vi "ReCalc_V0.14.vi"(3 "Berechnen":bool, 4 "Datenspeicher":T2) -> ()   [LabVIEW 2014]
uses:
  <vilib>/Utility/miscctls.llb/LVPointTypeDef.ctl
  <vilib>/Analysis/NI_AALBase.lvlib
  <vilib>/Analysis/NI_AALPro.lvlib
  <vilib>/Utility/xml.llb/Read From XML File(string).vi
  <vilib>/Analysis/3filter.llb/IIR Filter (DBL).vi
  <vilib>/Utility/xml.llb/Write to XML File(string).vi
panel:
  out "Fahrzeugdaten":string
  out "Überlagerung":bool
  in  "Überlagern":bool
  out "Übersetzung ermitteln aus":T1(ring)
  in  "Speichern":bool
  out "Reifenumfang [m]":dbl=1.222
  out "Getriebe [1:]":dbl=5.343
  out "Zündung [Imp/U]":u8=1
  out "Rolle [Inkr/U]":u16=200
  out "Luftdruck [mbar]":dbl=1013.0
  out "Luftfeuchtigkeit [%]":dbl=50.0
  out "Lufttemperatur [°C]":dbl=20.0
  in  "Stopp":bool
  in  "Rollenträgheit [kgm²]":dbl=0.402
  in  "Polynom":u8=15
  in  "Gl. Mittelwert":u8=35
  in  "Differenzenquotient":u8=12
  in  "n vom Gas [1/min]":dbl=5000.0
  out "Rollenumfang [m]":dbl=0.613 format="%.3f"
  out "Datum, Zeit":string
  out "Untersetzung aus:":dbl=2.68 format="%.2f"
  in  "Drucken":bool
  out "Pmax":string
  out "Ergebnis":string
  out "XY-Graph":cluster{dbl[], dbl[]}[](graph)
  in  "Öffnen":bool
  out "korr":dbl
  out "[s]":dbl=5.0
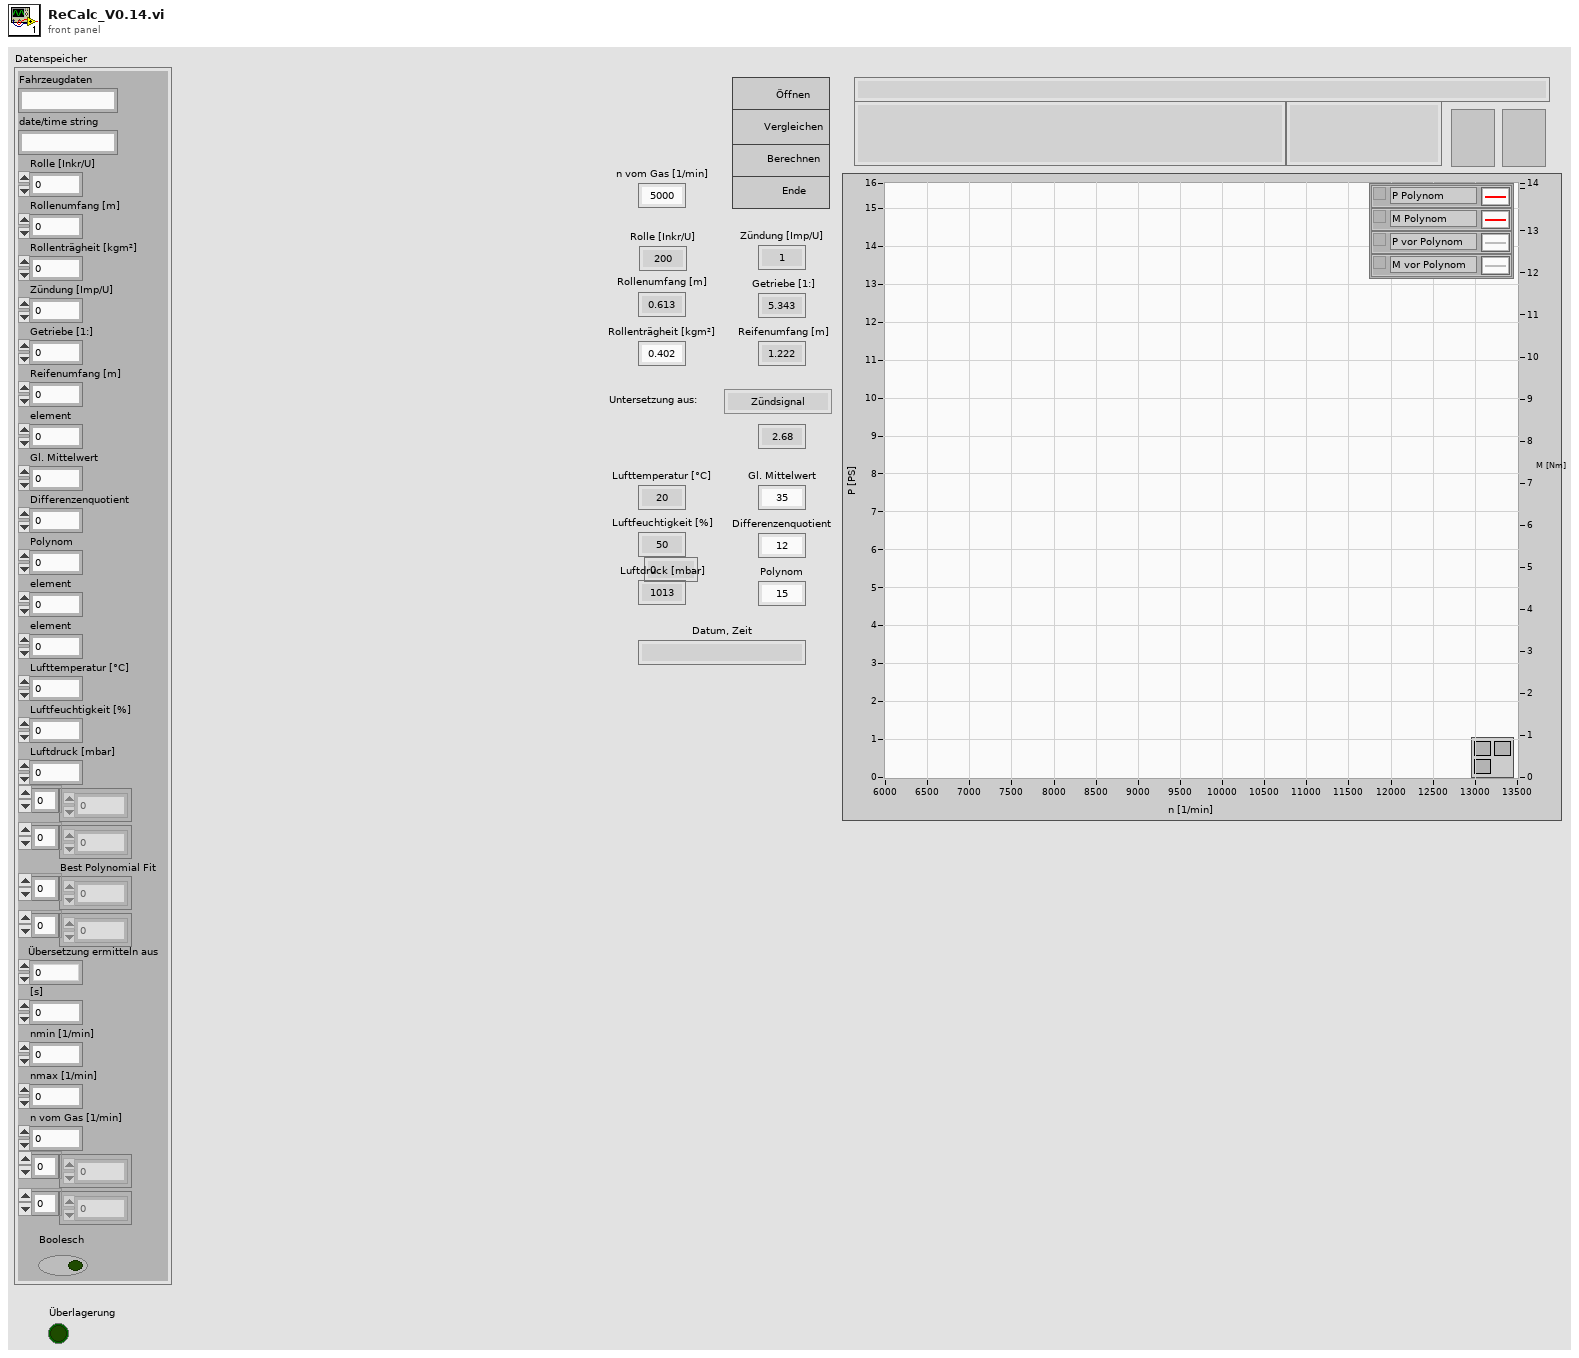
[diagram p1: front panel]
types:
  T1 = enum8{"Zündsignal", "Getriebe & Reifen", "nKuWe / nRolle :"}
  T2 = cluster{"Fahrzeugdaten":string, "date/time string":string, "Rolle [Inkr/U]":u16, "Rollenumfang [m]":dbl, "Rollenträgheit [kgm²]":dbl, "Zündung [Imp/U]":u8, "Getriebe [1:]":dbl, "Reifenumfang [m] ":dbl, "element":dbl, "Gl. Mittelwert":u8, "Differenzenquotient":u8, "Polynom":u8, "element":dbl, "element":dbl, "Lufttemperatur [°C]":dbl, "Luftfeuchtigkeit [%]":dbl, "Luftdruck [mbar]":dbl, dbl[], dbl[], "Best Polynomial Fit":dbl[], dbl[], "Übersetzung ermitteln aus":u8, "[s]":dbl, "nmin [1/min]":dbl, "nmax [1/min]":dbl, "n vom Gas [1/min]":dbl, dbl[], i32[], "Boolesch":bool}
  T3 = typedef "LVPointTypeDef.ctl" = cluster{"Horizontal":i16, "Vertical":i16}
  T4 = enum16{"Kleinste Quadrate", "Kleinestes absolutes Reiduum", "Biquadrat"}
  T5 = enum8{"Enabled", "Disabled", "Disabled and Grayed Out"}
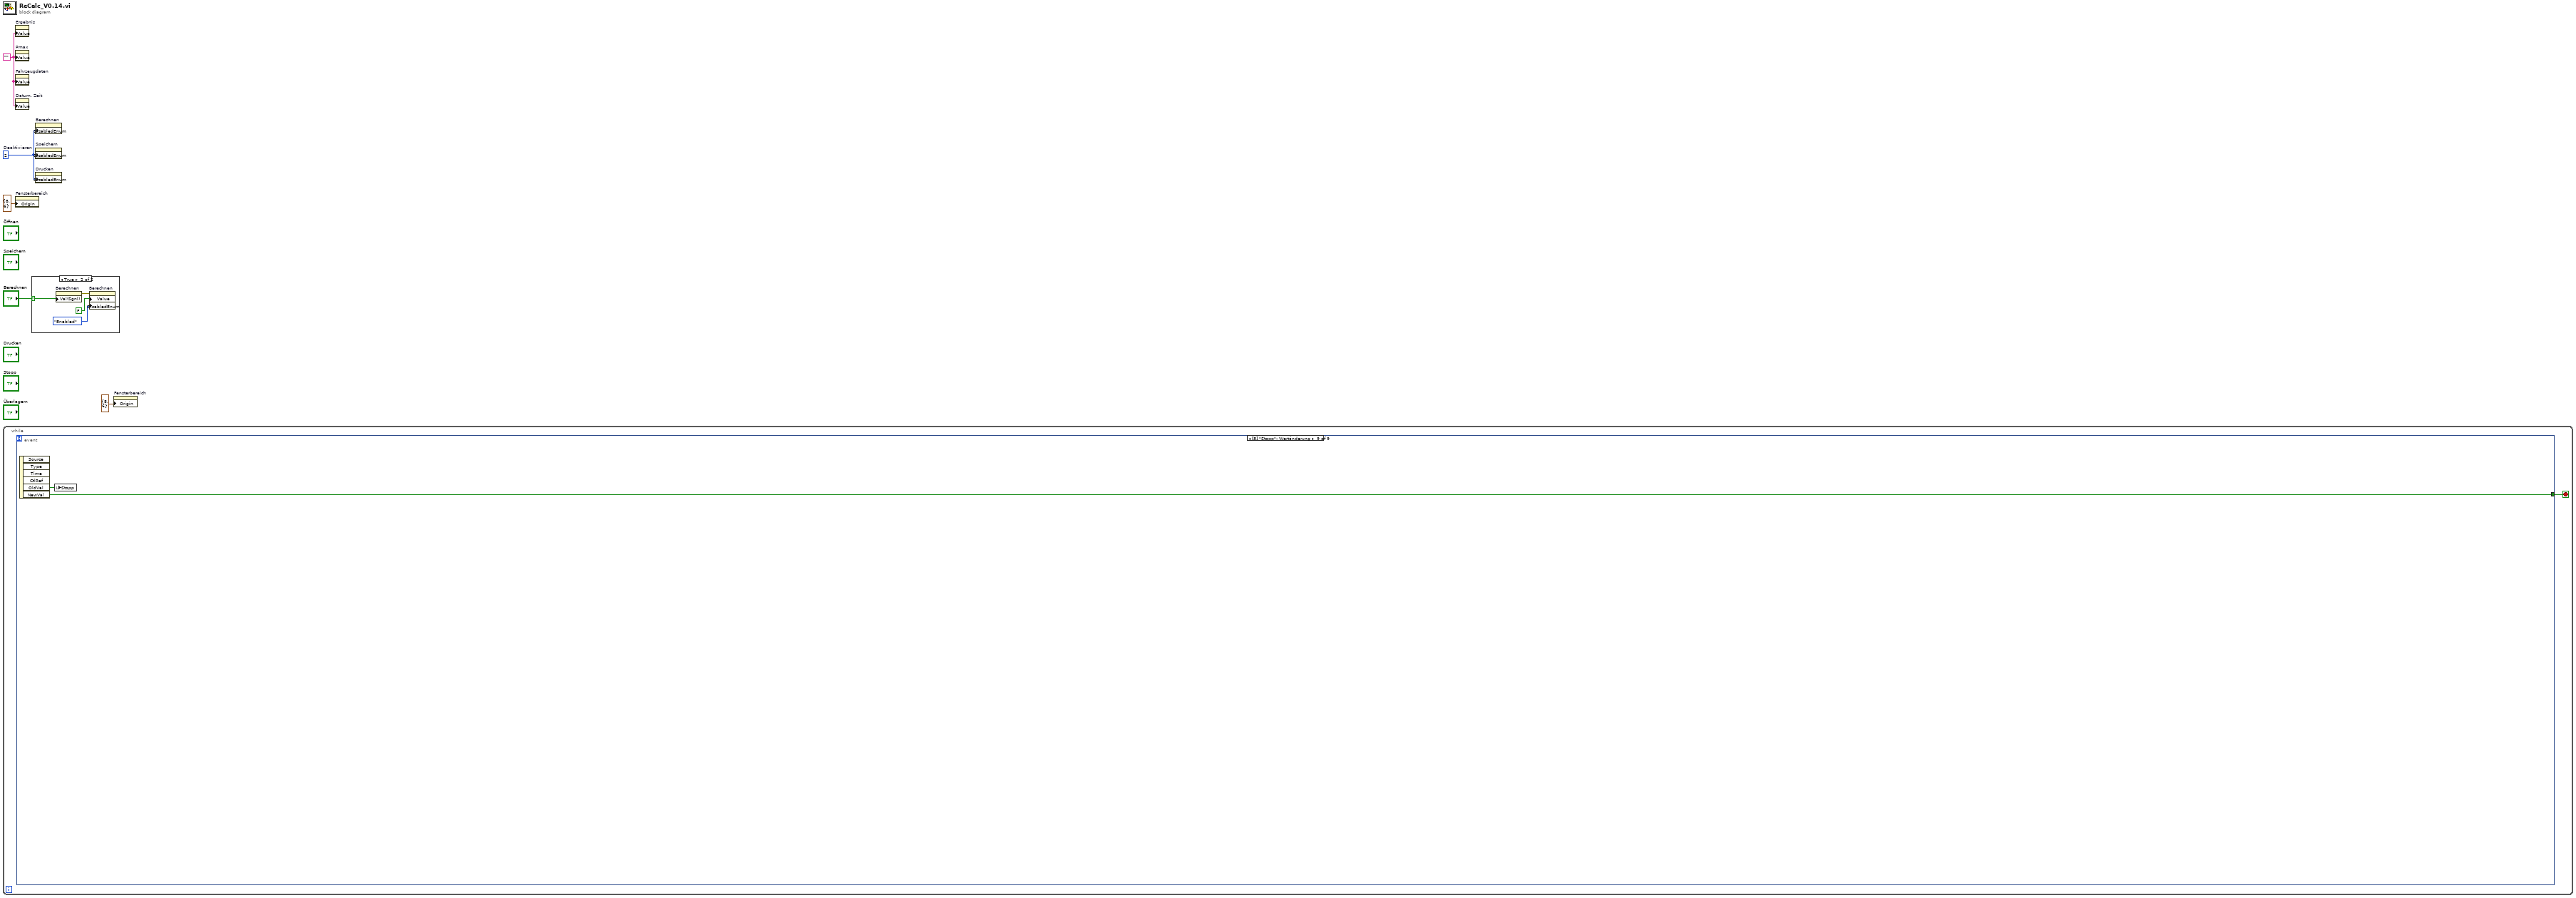
[diagram p0: block diagram]
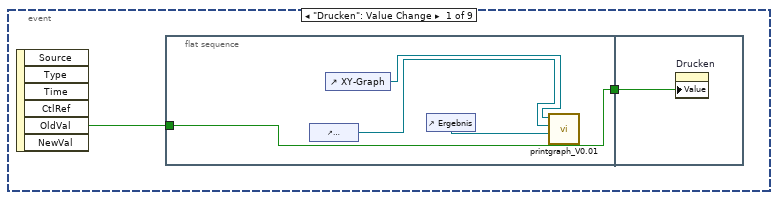
[diagram p3: hidden frame]
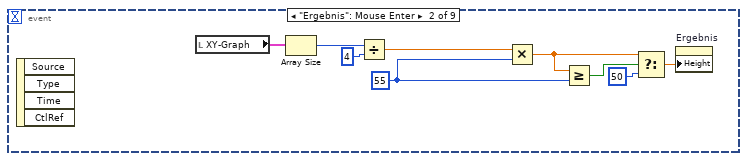
[diagram p4: hidden frame]
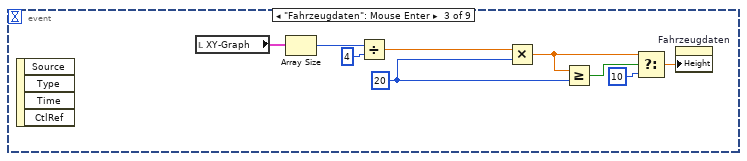
[diagram p5: hidden frame]
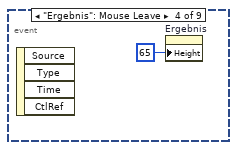
[diagram p6: hidden frame]
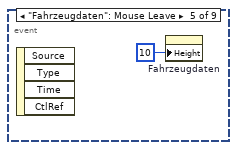
[diagram p7: hidden frame]
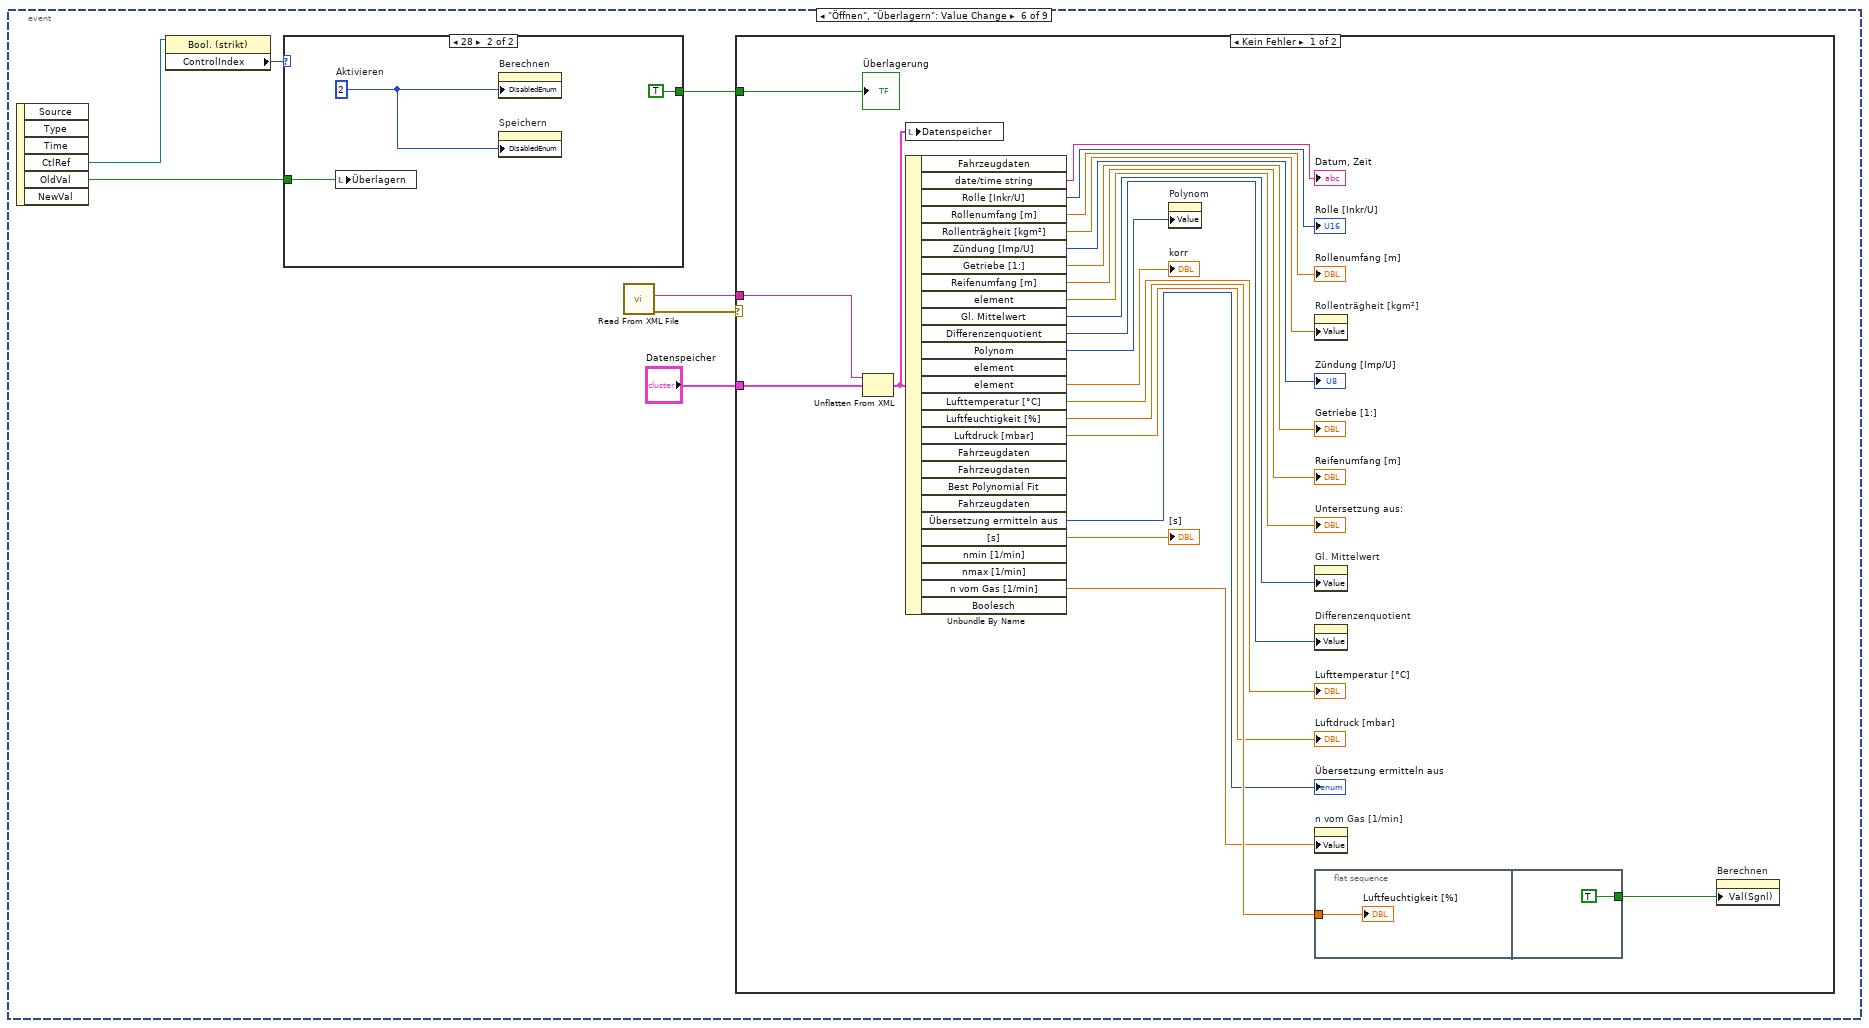
[diagram p8: hidden frame]
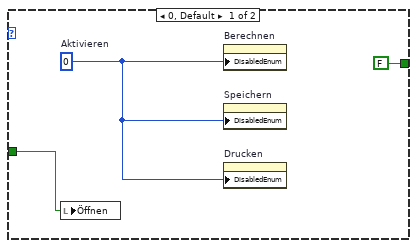
[diagram p9: hidden frame]
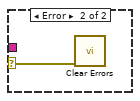
[diagram p10: hidden frame]
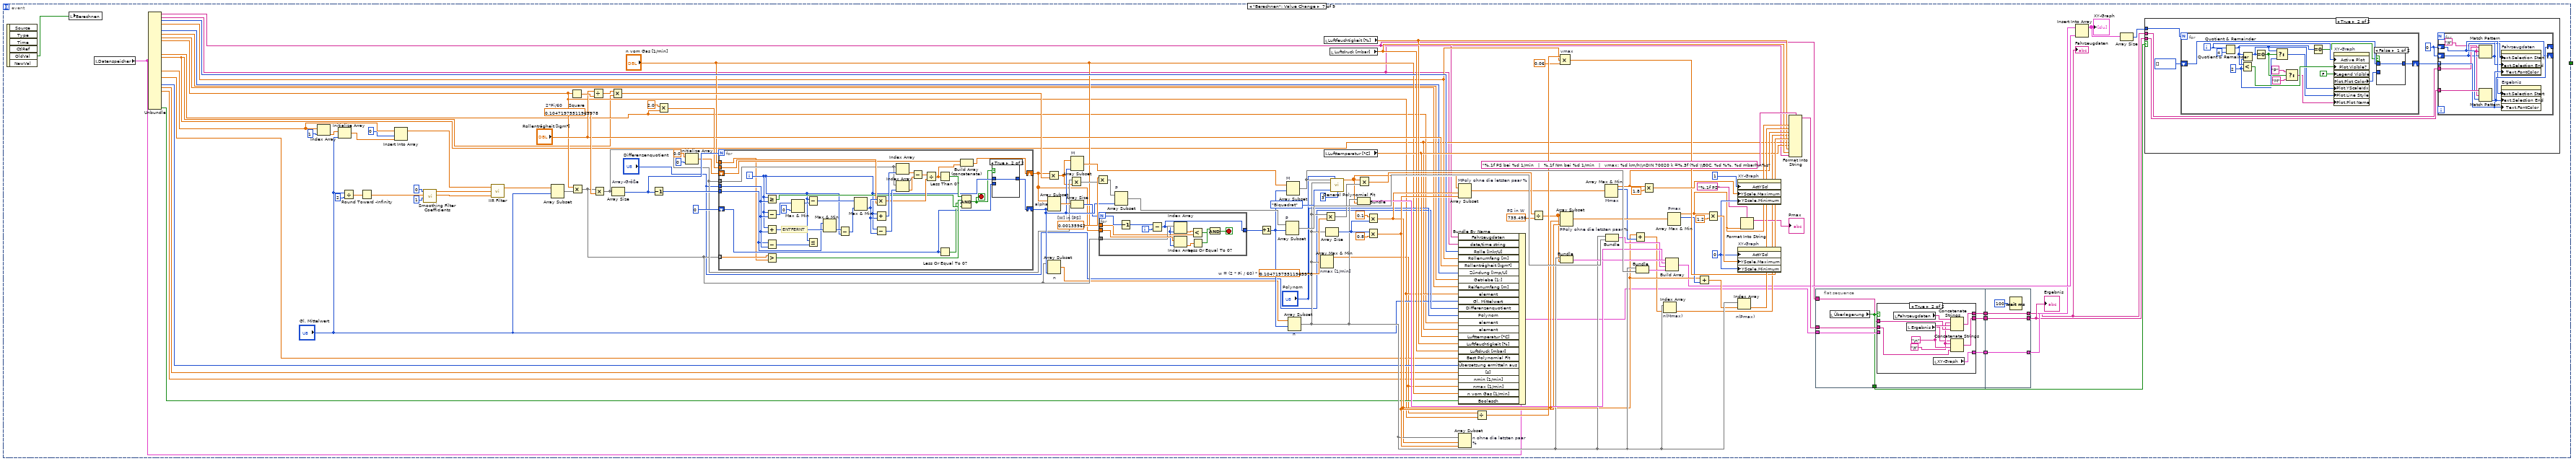
[diagram p11: hidden frame]
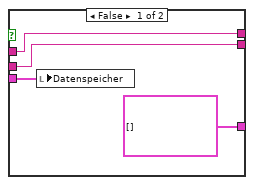
[diagram p12: hidden frame]
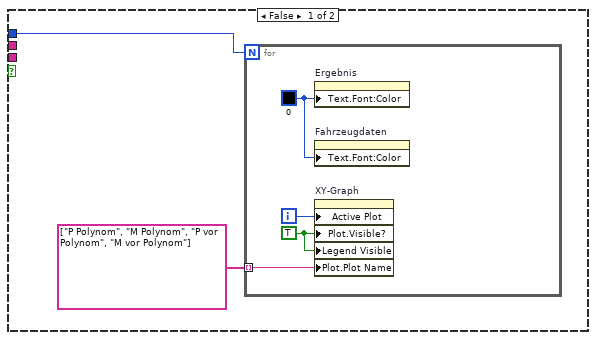
[diagram p13: hidden frame]
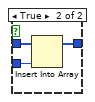
[diagram p14: hidden frame]
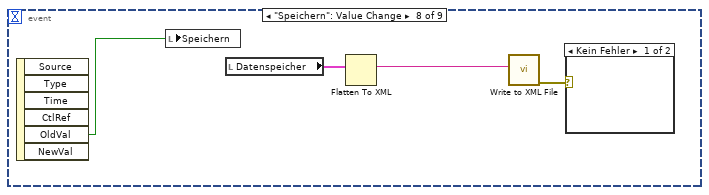
[diagram p16: hidden frame]
diagram:
  w3 = 2  # Deaktivieren
  w5 = ""
  n1 = while {
    stop <- w6 stop-if-true
    n2 = event shown="[8] \"Stopp\": Wertänderung" {
      selector: _ -> [_ _ _ _ _ _ _ _ _]
      dyn-events: _ -> [_ _ _ _ _ _ _ _ _]
      timeout: _ -> [_ _ _ _ _ _ _ _ _]
      tunnel: [_ _ _ _ _ _ _ _ w310] -> w6
      event "Drucken": Value Change {
        n3 = event-data() -> ("OldVal"=w8:bool)  [unwired: 1 in, 5 out]
        n4 = flat-sequence {
          tunnel: w8 -> [w12]
          tunnel: [w12] -> w7
          tunnel: w7 -> [w13]
          frame #0 {
            n5 = control-ref of="Fahrzeugdaten"() -> (w10:refnum<vi>)
            n6 = control-ref of="XY-Graph"() -> (w11:refnum<vi>)
            n7 = control-ref of="Ergebnis"() -> (w9:refnum<vi>)
            n8 = call "printgraph_V0.01.vi"("reference 2"=w9, "Fahrzeugdaten"=w10, "XYGraph (Eingang)"=w11) -> ()  [unwired: 9 in]
          }
          frame #1 {
            n9 = property on="Drucken" class="Bool. (strikt)"("Value"=w13) -> ()  [unwired: 2 in, 2 out]
          }
        }
      }
      event "Ergebnis": Mouse Enter {
        w16 = u32 55 ("Größe:Höhe")
        n10 = event-data() -> ()  [unwired: 1 in, 4 out]
        n11 = local read "XY-Graph"() -> (w22:cluster{dbl[], dbl[]}[])
        n12 = Array Size(array=w22) -> (size(s)=w21:i32)
        n13 = Divide(x=w21, y=4) -> (x/y=w19:dbl)
        n14 = Multiply(x=w19, y=w16) -> (x*y=w17:dbl)
        n15 = Greater Or Equal?(x=w17, y=w16) -> (x >= y?=w18:bool)
        n16 = Select(t=w17, s=w18, f=u32 50 ("Größe:Höhe")) -> (s? t:f=w15:dbl)
        n17 = property on="Ergebnis" class="Str"("Height"=w15) -> ()  [unwired: 2 in, 2 out]
      }
      event "Fahrzeugdaten": Mouse Enter {
        w25 = u32 20 ("Größe:Höhe")
        n18 = event-data() -> ()  [unwired: 1 in, 4 out]
        n19 = local read "XY-Graph"() -> (w31:cluster{dbl[], dbl[]}[])
        n20 = Array Size(array=w31) -> (size(s)=w30:i32)
        n21 = Divide(x=w30, y=4) -> (x/y=w28:dbl)
        n22 = Multiply(x=w28, y=w25) -> (x*y=w26:dbl)
        n23 = Greater Or Equal?(x=w26, y=w25) -> (x >= y?=w27:bool)
        n24 = Select(t=w26, s=w27, f=u32 10 ("Größe:Höhe")) -> (s? t:f=w24:dbl)
        n25 = property on="Fahrzeugdaten" class="Str"("Height"=w24) -> ()  [unwired: 2 in, 2 out]
      }
      event "Ergebnis": Mouse Leave {
        n26 = event-data() -> ()  [unwired: 1 in, 4 out]
        n27 = property on="Ergebnis" class="Str"("Height"=u32 65 ("Größe:Höhe")) -> ()  [unwired: 2 in, 2 out]
      }
      event "Fahrzeugdaten": Mouse Leave {
        n28 = event-data() -> ()  [unwired: 1 in, 4 out]
        n29 = property on="Fahrzeugdaten" class="Str"("Height"=u32 10 ("Größe:Höhe")) -> ()  [unwired: 2 in, 2 out]
      }
      event "Öffnen", "Überlagern": Value Change {
        n30 = event-data() -> ("CtlRef"=w37:refnum<vi>, "OldVal"=w35:bool)  [unwired: 1 in, 4 out]
        n31 = property class="Bool. (strikt)"(reference=w37) -> ("ControlIndex"=w36:i32)  [unwired: 1 in, 2 out]
        n32 = case shown="28" w36 {
          tunnel: w35 -> [w43 w46]
          tunnel: [FALSE ("Überlagerung") TRUE ("Überlagerung")] -> w34
          frame 0, Default {
            w41 = 0  # Aktivieren
            n33 = local write "Öffnen"(w43) -> ()
            n34 = property on="Berechnen" class="Bool. (strikt)"("DisabledEnum"=w41) -> ()  [unwired: 2 in, 2 out]
            n35 = property on="Speichern" class="Bool. (strikt)"("DisabledEnum"=w41) -> ()  [unwired: 2 in, 2 out]
            n36 = property on="Drucken" class="Bool. (strikt)"("DisabledEnum"=w41) -> ()  [unwired: 2 in, 2 out]
          }
          frame 28 {
            w44 = 2  # Aktivieren
            n37 = local write "Überlagern"(w46) -> ()
            n38 = property on="Berechnen" class="Bool. (strikt)"("DisabledEnum"=w44) -> ()  [unwired: 2 in, 2 out]
            n39 = property on="Speichern" class="Bool. (strikt)"("DisabledEnum"=w44) -> ()  [unwired: 2 in, 2 out]
          }
        }
        n40 = call-poly <vilib>:"Read From XML File.vi"() -> ("error out"=w38:errorcluster, "XML Elements"=w40:string)  [unwired: 9 in, 1 out]
        n41 = case shown="Kein Fehler" w38 {
          selector: w38 -> [_ w72]
          tunnel: w40 -> [w69 _]
          tunnel: "Datenspeicher" -> [w68 _]
          tunnel: w34 -> [w48 _]
          frame No Error {
            n42 = Unflatten From XML(xml string=w69, type=w68) -> (value=w49:T2)  [unwired: 1 in, 1 out]
            n43 = local write "Datenspeicher"(w49) -> ()
            n44 = Unbundle By Name(w49) -> ("date/time string"=→"Datum, Zeit":string, "Rolle [Inkr/U]"=→"Rolle [Inkr/U]":u16, "Rollenumfang [m]"=→"Rollenumfang [m]":dbl, "Rollenträgheit [kgm²]"=w64:dbl, "Zündung [Imp/U]"=→"Zündung [Imp/U]":u8, "Getriebe [1:]"=→"Getriebe [1:]":dbl, "Reifenumfang [m]"=→"Reifenumfang [m]":dbl, "element"=→"Untersetzung aus:":dbl, "Gl. Mittelwert"=w61:u8, "Differenzenquotient"=w60:u8, "Polynom"=w59:u8, "element"=→"korr":dbl, "Lufttemperatur [°C]"=→"Lufttemperatur [°C]":dbl, "Luftfeuchtigkeit [%]"=w57:dbl, "Luftdruck [mbar]"=→"Luftdruck [mbar]":dbl, "Übersetzung ermitteln aus"=→"Übersetzung ermitteln aus":u8, "[s]"=→"[s]":dbl, "n vom Gas [1/min]"=w52:dbl)  [unwired: 9 out]
            n45 = property on="Polynom" class="DigWert (strikt)"("Value"=w59) -> ()  [unwired: 2 in, 2 out]
            n46 = property on="Rollenträgheit [kgm²]" class="DigWert (strikt)"("Value"=w64) -> ()  [unwired: 2 in, 2 out]
            n47 = property on="Gl. Mittelwert" class="DigWert (strikt)"("Value"=w61) -> ()  [unwired: 2 in, 2 out]
            n48 = property on="Differenzenquotient" class="DigWert (strikt)"("Value"=w60) -> ()  [unwired: 2 in, 2 out]
            n49 = property on="n vom Gas [1/min]" class="DigWert (strikt)"("Value"=w52) -> ()  [unwired: 2 in, 2 out]
            n50 = flat-sequence {
              tunnel: w57 -> [w70]
              tunnel: [TRUE] -> w50
              frame #0 {
                "Luftfeuchtigkeit [%]" <- w70
              }
              frame #1 {
              }
            }
            n51 = property on="Berechnen" class="Bool. (strikt)"("Val(Sgnl)"=w50) -> ()  [unwired: 2 in, 2 out]
            "Überlagerung" <- w48
          }
          frame Error {
            n52 = call <vilib>:"Clear Errors.vi"("error in (no error)"=w72) -> ()  [unwired: 5 in, 2 out]
          }
        }
      }
      event "Berechnen": Value Change {
        w155 = 0
        w163 = 735.498  # PS in W
        w168 = 0.10471975511965978  # w = (2 * Pi / 60) * n
        w179 = 0.00135962  # [W] in [PS]
        w188 = 0.10471975511965978  # 2*Pi/60
        n53 = event-data() -> ("OldVal"=w85:bool)  [unwired: 1 in, 5 out]
        n54 = local write "Berechnen"(w85) -> ()
        n55 = local read "Datenspeicher"() -> (w111:T2)
        n56 = Unbundle(w111) -> ("Fahrzeugdaten"=w77:string, "date/time string"=w76:string, "Rolle [Inkr/U]"=w107:u16, "Rollenumfang [m]"=w98:dbl, "Zündung [Imp/U]"=w97:u8, "Getriebe [1:]"=w96:dbl, "Reifenumfang [m]"=w95:dbl, "element"=w94:dbl, "element"=w93:dbl, "element"=w92:dbl, w194:dbl[], "Best Polynomial Fit"=w91:dbl[], "Übersetzung ermitteln aus"=w99:u8, "[s]"=w88:dbl, "nmin [1/min]"=w89:dbl, "Boolesch"=w102:bool)  [unwired: 13 out]
        n57 = Index Array(array=w194, index=1) -> (element=w117:dbl)
        n58 = Initialize Array(w117, "Gl. Mittelwert") -> (w118:dbl[])
        n59 = Divide(x="Gl. Mittelwert", y=2) -> (x/y=w191:dbl)
        n60 = Round Toward -Infinity(1:w191) -> (0:w190:dbl)
        n61 = Insert Into Array ("In Array einfügen")(array=w194, index=0, new element=w118) -> (w115:dbl[])
        n62 = call <vilib>:"Smoothing Filter Coefficients.vi"("shape"=1, "half-width"=w190, "type"=0) -> ("forward coefficients"=w119:dbl[], "reverse coefficients"=w120:dbl[])  [unwired: 6 in, 1 out]
        n63 = call-poly <vilib>:"IIR Filter.vi"("Forward Coefficients"=w119, "Reverse Coefficients"=w120, "X"=w115) -> ("Filtered X"=w114:dbl[])  [unwired: 1 in, 1 out]
        n64 = Array Subset(array=w114, index="Gl. Mittelwert") -> (w113:dbl[])  [unwired: 1 in]
        n65 = Square(x=w94) -> (x^2=w180:dbl)
        n66 = Multiply(x=w94, y=w113) -> (x*y=w122:dbl[])
        n67 = Divide(x="Rollenträgheit [kgm²]", y=w180) -> (x/y=w177:dbl)
        n68 = Multiply(x=w122, y=w188) -> (x*y=w145:dbl[])
        n69 = Multiply(x=w177, y=w92) -> (x*y=w176:dbl)
        n70 = Array Size "Array-Größe"(array=w145) -> (size(s)=w186:i32)
        n71 = Decrement(x=w186) -> (x-1=w187:i32)
        n72 = Multiply(x=2.0, y=w93) -> (x*y=w185:dbl)
        n73 = Initialize Array(0.0 ("y"), 0) -> (w181:dbl[])
        n74 = for {
          N: w186 -> [_]
          tunnel: "Differenzenquotient" -> [w281]
          tunnel: w145 -> [w288]
          tunnel: w187 -> [w280]
          tunnel: w185 -> [w289]
          shift-right: [w285] -> w144
          shift-left: w181 -> [w286]
          tunnel: w122 -> [w283] mode=indexing
          tunnel: "n vom Gas [1/min]" -> [w272]
          shift-right: [w271] -> w172
          shift-left: 0 -> [w274]
          i -> [w275]
          stop <- w273 stop-if-true
          # "ENTFERNT"
          n75 = Greater Or Equal?(x=w275, y=w281) -> (x >= y?=w278:bool)
          n76 = Subtract(x=w275, y=w281) -> (x-y=w302:i32)
          n77 = Add(x=w275, y=w281) -> (x+y=w296:i32)
          n78 = Subtract(x=w280, y=w281) -> (x-y=w282:i32)
          n79 = Greater?(x=w283, y=w272) -> (0:w284:bool)
          n80 = Max & Min(x=w302, y=0) -> (max(x,y)=w300:i32)  [unwired: 1 out]
          n81 = Subtract(x=w275, y=w300) -> (x-y=w299:i32)
          n82 = Less Or Equal?(x=w275, y=w282) -> ()  [unwired: 1 out]
          n83 = Max & Min(x=w280, y=w296) -> (min(x,y)=w297:i32)  [unwired: 1 out]
          n84 = Subtract(x=w297, y=w275) -> (x-y=w298:i32)
          n85 = Max & Min(x=w299, y=w298) -> (min(x,y)=w290:i32)  [unwired: 1 out]
          n86 = Multiply(x=w290, y=w289) -> (x*y=w287:dbl)
          n87 = Add(x=w275, y=w290) -> (x+y=w295:i32)
          n88 = Subtract(x=w275, y=w290) -> (x-y=w294:i32)
          n89 = Index Array(array=w288, index=w295) -> (element=w292:dbl)
          n90 = Index Array(array=w288, index=w294) -> (element=w293:dbl)
          n91 = Subtract(x=w292, y=w293) -> (x-y=w291:dbl)
          n92 = Divide(x=w291, y=w287) -> (x/y=w279:dbl)
          n93 = Less Than 0?(x=w279) -> (x < 0?=w277:bool)
          n94 = Less Or Equal To 0?(x=w274) -> (x <= 0?=w276:bool)
          n95 = Build Array (concatenate)(w286, w279) -> (w285:dbl[])
          n96 = Compound Arithmetic op=AND(w277, w284, w276, w278) -> (w273:bool)
          n97 = case shown="True" w273 {
            tunnel: w275 -> [_ w304]
            tunnel: [w303 w304] -> w271
            tunnel: w274 -> [w303 _]
            frame False {
            }
            frame True {
            }
          }
        }
        n98 = Multiply(x=w144, y=w176) -> (x*y=w142:dbl[])
        n99 = Array Subset "alpha"(array=w144, length=w172) -> (w174:dbl[])  [unwired: 1 in]
        n100 = Array Subset "n"(array=w122, length=w172) -> (w121:dbl[])  [unwired: 1 in]
        n101 = Multiply(x=w145, y=w142) -> (x*y=w178:dbl[])
        n102 = Array Subset "M"(array=w142, length=w172) -> (w143:dbl[])  [unwired: 1 in]
        n103 = Array Size(array=w174) -> (size(s)=w171:i32)
        n104 = Multiply(x=w179, y=w178) -> (x*y=w173:dbl[])
        n105 = for {
          N: w171 -> [w270]
          tunnel: w144 -> [w267]
          tunnel: w122 -> [w264]
          tunnel: "n vom Gas [1/min]" -> [w261]
          tunnel: [w259] -> w170
          i -> [w265]
          stop <- w260 stop-if-true
          n106 = Decrement(x=w270) -> (x-1=w269:i32)
          n107 = Subtract(x=w269, y=w265) -> (x-y=w259:i32)
          n108 = Index Array(array=w264, index=w259) -> (element=w263:dbl)
          n109 = Index Array(array=w267, index=w259) -> (element=w268:dbl)
          n110 = Less?(x=w263, y=w261) -> (x < y?=w262:bool)
          n111 = Less Or Equal To 0?(x=w268) -> (x <= 0?=w266:bool)
          n112 = And(x=w266, y=w262) -> (x .and. y?=w260:bool)
        }
        n113 = Array Subset "P"(array=w173, length=w172) -> (w162:dbl[])  [unwired: 1 in]
        n114 = Increment(x=w170) -> (x+1=w161:i32)
        n115 = Array Subset "P"(array=w162, index=w161) -> (w169:dbl[])  [unwired: 1 in]
        n116 = Array Subset "M"(array=w143, index=w161) -> (w167:dbl[])  [unwired: 1 in]
        n117 = Array Subset "n"(array=w121, index=w161) -> (w130:dbl[])  [unwired: 1 in]
        n118 = Array Max & Min "nmax [1/min]"(array=w130) -> (max value=w90:dbl)  [unwired: 3 out]
        n119 = local read "Luftfeuchtigkeit [%]"() -> (w109:dbl)
        n120 = local read "Lufttemperatur [°C]"() -> (w108:dbl)
        n121 = Multiply(x=w130, y=w168) -> (x*y=w154:dbl[])
        n122 = Array Size(array=w130) -> (size(s)=w132:i32)
        n123 = local read "Luftdruck [mbar]"() -> (w110:dbl)
        n124 = call <vilib>:"General Polynomial Fit.vi"("Y"=w167, "polynomial order"="Polynom", "X"=w130, "method"=T4."Biquadrat" ("Methode"), "algorithm"=3) -> ("Best Polynomial Fit"=w129:dbl[])  [unwired: 7 in, 3 out]
        n125 = Bundle(w130, "Best Polynomial Fit"=w129) -> (w140:cluster{dbl[], "Best Polynomial Fit":dbl[]})  [unwired: 1 in]
        n126 = Multiply(x=w129, y=w154) -> (x*y=w164:dbl[])
        n127 = Multiply(x=0.1, y=w132) -> (x*y=w125:dbl)
        n128 = Multiply(x=w132, y=0.8) -> (x*y=w133:dbl)
        n129 = Array Subset "MPoly ohne die letzten paar %"(array=w129, index=w125, length=w133) -> (w134:dbl[])
        n130 = Bundle By Name(cluster=w111, "Fahrzeugdaten"=w77, "date/time string"=w76, "Rolle [Inkr/U]"=w107, "Rollenumfang [m]"=w98, "Rollenträgheit [kgm²]"="Rollenträgheit [kgm²]", "Zündung [Imp/U]"=w97, "Getriebe [1:]"=w96, "Reifenumfang [m]"=w95, "element"=w94, "Gl. Mittelwert"="Gl. Mittelwert", "Differenzenquotient"="Differenzenquotient", "Polynom"="Polynom", "element"=w93, "element"=w92, "Lufttemperatur [°C]"=w108, "Luftfeuchtigkeit [%]"=w109, "Luftdruck [mbar]"=w110, "Best Polynomial Fit"=w91, "Übersetzung ermitteln aus"=w99, "[s]"=w88, "nmin [1/min]"=w89, "nmax [1/min]"=w90, "n vom Gas [1/min]"="n vom Gas [1/min]", "Boolesch"=w102) -> (w83:T2)
        n131 = Array Subset "n ohne die letzten paar %"(array=w130, index=w125, length=w133) -> ()  [unwired: 1 out]
        n132 = Divide(x=w90, y=w94) -> (x/y=w153:dbl)
        n133 = Divide(x=w164, y=w163) -> (x/y=w128:dbl[])
        n134 = Compound Arithmetic op=MULTIPLY "vmax"(w153, w98, 0.06) -> (w150:dbl)
        n135 = Array Subset "PPoly ohne die letzten paar %"(array=w128, index=w125, length=w133) -> (w135:dbl[])
        n136 = Bundle(w130, w128) -> (w141:cluster{dbl[], dbl[]})  [unwired: 1 in]
        n137 = Array Max & Min "Mmax"(array=w134) -> (max value=w147:dbl, max index (indices)=w126:i32)  [unwired: 2 out]
        n138 = Bundle(w130, w169) -> (w139:cluster{dbl[], dbl[]})  [unwired: 1 in]
        n139 = Add(x=w125, y=w126) -> (x+y=w124:dbl)
        n140 = Bundle(w130, w167) -> (w138:cluster{dbl[], dbl[]})  [unwired: 1 in]
        n141 = Multiply(x=w147, y=1.8) -> (x*y=w156:dbl)
        n142 = Index Array "n(Mmax)"(array=w130, index=w124) -> (element=w100:dbl)
        n143 = Build Array(w141, w140, w139, w138) -> (w81:cluster{dbl[], "Best Polynomial Fit":dbl[]}[])
        n144 = Array Max & Min "Pmax"(array=w135) -> (max value=w148:dbl, max index (indices)=w127:i32)  [unwired: 2 out]
        n145 = Add(x=w125, y=w127) -> (x+y=w123:dbl)
        n146 = Multiply(x=w148, y=1.2) -> (x*y=w157:dbl)
        n147 = property on="XY-Graph" class="XYGraph (strikt)"("ActYScl"=1, "YScale.Maximum"=w156, "YScale.Minimum"=w155) -> ()  [unwired: 2 in, 2 out]
        n148 = property on="XY-Graph" class="XYGraph (strikt)"("ActYScl"=w155, "YScale.Maximum"=w157, "YScale.Minimum"=w155) -> ()  [unwired: 2 in, 2 out]
        n149 = Index Array "n(Pmax)"(array=w130, index=w123) -> (element=w151:dbl)
        n150 = Format Into String(format string="%.1f PS" ("Format-String"), w148) -> (resulting string=→"Pmax":string)  [unwired: 2 in, 1 out]
        n151 = Format Into String(format string="%.1f PS bei %d 1/min   |   %.1f Nm bei %d 1/min   |   vmax: %d km/h\\nDIN 70020 k =%.3f (%d \\B0C, %d %%, %d mbar)\\n%s" ("Format-String"), w148, w151, w147, w100, w150, w92, w108, w109, w110, w76) -> (resulting string=w87:string)  [unwired: 2 in, 1 out]
        n152 = flat-sequence {
          tunnel: w87 -> [w201]
          tunnel: w83 -> [w200]
          tunnel: [w199] -> w82
          tunnel: w77 -> [w195]
          tunnel: [w198] -> w75
          tunnel: [w197] -> w74
          tunnel: [w196] -> w73
          tunnel: [w216] -> w78
          tunnel: [w217] -> w79
          tunnel: [w218] -> w80
          tunnel: w75 -> [w218]
          tunnel: w74 -> [w217]
          tunnel: w73 -> [w216]
          frame #0 {
            n153 = local read "Überlagerung"() -> (w199:bool)
            n154 = case shown="True" w199 {
              tunnel: [cluster{dbl[], dbl[]}[] [] ("XY-Graph") w214] -> w198
              tunnel: w201 -> [w204 w212]
              tunnel: [w204 w213] -> w197
              tunnel: w200 -> [w203 _]
              tunnel: w195 -> [w202 w210]
              tunnel: [w202 w209] -> w196
              frame False {
                n155 = local write "Datenspeicher"(w203) -> ()
              }
              frame True {
                w208 = "\t"
                w211 = "\n"
                n156 = local read "Fahrzeugdaten"() -> (w207:string)
                n157 = local read "Ergebnis"() -> (w206:string)
                n158 = local read "XY-Graph"() -> (w214:cluster{dbl[], dbl[]}[])
                n159 = Concatenate Strings(w207, w208, w211, w210) -> (w209:string)
                n160 = Concatenate Strings(w206, w208, w211, w212) -> (w213:string)
              }
            }
          }
          frame #1 {
            n161 = Wait (ms)(milliseconds to wait=u32 100 ("Zu wartende ms")) -> ()  [unwired: 1 out]
          }
        }
        n162 = Insert Into Array(array=w80, new element=w81) -> (w84:cluster{dbl[], dbl[]}[])  [unwired: 1 in]
        "XY-Graph" <- w84
        n163 = Array Size(array=w84) -> (size(s)=w86:i32)
        n164 = case shown="True" w82 {
          tunnel: w86 -> [w220 w230]
          tunnel: w79 -> [_ w227]
          tunnel: w78 -> [_ w226]
          frame False {
            n165 = for {
              N: w220 -> [_]
              tunnel: string[] ["P Polynom", "M Polynom", "P vor Polynom", "M vor Polynom"] -> [w222] mode=indexing
              i -> [w224]
              w221 = u32 0
              w223 = TRUE ("Plot.Sichtbar")
              n166 = property on="Ergebnis" class="Str"("Text.Font:Color"=w221) -> ()  [unwired: 2 in, 2 out]
              n167 = property on="Fahrzeugdaten" class="Str"("Text.Font:Color"=w221) -> ()  [unwired: 2 in, 2 out]
              n168 = property on="XY-Graph" class="XYGraph (strikt)"("Active Plot"=w224, "Plot.Visible?"=w223, "Legend Visible"=w223, "Plot.Plot Name"=w222) -> ()  [unwired: 2 in, 2 out]
            }
          }
          frame True {
            w225 = 0
            n169 = for {
              N: w230 -> [_]
              shift-right: [w249] -> w228
              shift-left: u32[] [] -> [w248]
              i -> [w253]
              w244 = 2 ("y")
              n170 = Quotient & Remainder(x=w253, y=4) -> (x-y*floor(x/y)=w246:i32)  [unwired: 1 out]
              n171 = Less?(x=w246, y=w244) -> (x < y?=w252:bool)
              n172 = Quotient & Remainder(x=w246, y=w244) -> (x-y*floor(x/y)=w245:i32)  [unwired: 1 out]
              n173 = Equal To 0?(x=w245) -> (x = 0?=w242:bool)
              n174 = Select(t=w245, s=w242, f=w244) -> (s? t:f=w243:i32)
              n175 = Select(t="P" ("Plot.Plotname"), s=w242, f="M" ("Plot.Plotname")) -> (s? t:f=w239:string)
              n176 = Equal To 0?(x=w246) -> (x = 0?=w247:bool)
              n177 = property on="XY-Graph" class="XYGraph (strikt)"("Active Plot"=w253, "Plot.Visible?"=w252, "Legend Visible"=FALSE ("Legende:Sichtbar"), "Plot.YScaleIdx"=w245, "Plot.Line Style"=w243, "Plot.Plot Name"=w239) -> ("Plot.Plot Color"=w250:u32)  [unwired: 2 in, 2 out]
              n178 = case shown="False" w247 {
                tunnel: w250 -> [_ w258]
                tunnel: [w255 w257] -> w249
                tunnel: w248 -> [w255 w256]
                frame False {
                }
                frame True {
                  n179 = Insert Into Array(array=w256, new element=w258) -> (w257:u32[])  [unwired: 1 in]
                }
              }
            }
            n180 = for {
              shift-right: [w238] -> _
              shift-left: w225 -> [w235]
              tunnel: w228 -> [w236] mode=indexing
              tunnel: w227 -> [w237]
              tunnel: w226 -> [w234]
              shift-right: [w233] -> _
              shift-left: w225 -> [w232]
              w231 = "\t"
              n181 = Match Pattern(string=w234, regular expression=w231, offset (0)=w232) -> (offset past match=w233:i32)  [unwired: 3 out]
              n182 = Match Pattern(string=w237, regular expression=w231, offset (0)=w235) -> (offset past match=w238:i32)  [unwired: 3 out]
              n183 = property on="Fahrzeugdaten" class="Str"("Text.Selection Start"=w232, "Text.Selection End"=w233, "Text.FontColor"=w236) -> ()  [unwired: 2 in, 2 out]
              n184 = property on="Ergebnis" class="Str"("Text.Selection Start"=w235, "Text.Selection End"=w238, "Text.FontColor"=w236) -> ()  [unwired: 2 in, 2 out]
            }
          }
        }
        "Ergebnis" <- w79
        "Fahrzeugdaten" <- w78
      }
      event "Speichern": Value Change {
        n185 = event-data() -> ("OldVal"=w305:bool)  [unwired: 1 in, 5 out]
        n186 = local write "Speichern"(w305) -> ()
        n187 = local read "Datenspeicher"() -> (w306:T2)
        n188 = Flatten To XML(anything=w306) -> (xml string=w308:string)
        n189 = call-poly <vilib>:"Write to XML File.vi"("XML Input"=w308) -> ("error out"=w307:errorcluster)  [unwired: 8 in, 2 out]
        n190 = case shown="Kein Fehler" w307 {
          frame No Error {
          }
          frame Error {
          }
        }
      }
      event "Stopp": Value Change {
        n191 = event-data() -> ("OldVal"=w309:bool, "NewVal"=w310:bool)  [unwired: 1 in, 4 out]
        n192 = local write "Stopp"(w309) -> ()
      }
    }
  }
  n193 = property on="Ergebnis" class="Str"("Value"=w5) -> ()  [unwired: 2 in, 2 out]
  n194 = property on="Pmax" class="Str"("Value"=w5) -> ()  [unwired: 2 in, 2 out]
  n195 = property on="Fahrzeugdaten" class="Str"("Value"=w5) -> ()  [unwired: 2 in, 2 out]
  n196 = property on="Datum, Zeit" class="Str"("Value"=w5) -> ()  [unwired: 2 in, 2 out]
  n197 = property on="Fensterbereich" class="Bereich"("Origin"=T3 {"Horizontal"=8, "Vertical"=6}) -> ()  [unwired: 2 in, 2 out]
  n198 = case shown="True" "Berechnen" {
    selector: "Berechnen" -> [_ w314]
    frame False {
    }
    frame True {
      n199 = property on="Berechnen" class="Bool. (strikt)"("Val(Sgnl)"=w314) -> (error out=w313:errorcluster)  [unwired: 2 in, 1 out]
      n200 = property on="Berechnen" class="Bool. (strikt)"(error in=w313, "Value"=FALSE ("Berechnen"), "DisabledEnum"=T5."Enabled" ("Deaktiviert")) -> ()  [unwired: 1 in, 2 out]
    }
  }
  n201 = property on="Berechnen" class="Bool. (strikt)"("DisabledEnum"=w3) -> ()  [unwired: 2 in, 2 out]
  n202 = property on="Speichern" class="Bool. (strikt)"("DisabledEnum"=w3) -> ()  [unwired: 2 in, 2 out]
  n203 = property on="Drucken" class="Bool. (strikt)"("DisabledEnum"=w3) -> ()  [unwired: 2 in, 2 out]
  n204 = property on="Fensterbereich" class="Bereich"("Origin"=T3 {"Horizontal"=8, "Vertical"=6}) -> ()  [unwired: 2 in, 2 out]
